vi "Send Display Settings to Analyze Actor.vi"(8 "error in (no error)":errorcluster, 11 "AF IMAQ Display in":refnum<class "HIJ Vision Display.lvclass">) -> (0 "error out":errorcluster, 3 "AF IMAQ Display out":refnum<class "HIJ Vision Display.lvclass">)   [LabVIEW 2020, in "HIJ Vision Display.lvlib" / "HIJ Vision Display.lvclass"]
uses:
  HIJ Vision Display.lvclass
  HIJ Vision Display.lvclass/HIJ Vision Display.ctl
  Analyze/Analyze Parameter/Analyze Parameter Calibration/Analyze Parameter Calibration.lvclass
  C:/POLARIS Programme/POLARIS-AS-3-Cams/Submodules/HIJ Vision/Analyze/Analyze Parameter/Analyze Parameter Base/Analyze Parameter Base.lvclass
  Analyze/Analyze Parameter/Analyze Parameter ROI/Analyze Parameter ROI.lvclass
  Analyze/Analyze Parameter/Analyze Parameter ROI/Analyze Parameter ROI.lvclass/Analyze Parameter ROI.ctl
  Analyze/Analyze Actor/Analyze Actor Messages/Set Analyze Parameter Msg/Set Analyze Parameter Msg.lvclass/Set Analyze Parameter Msg.ctl
  <vilib>/ActorFramework/Message Enqueuer/Message Enqueuer.lvclass/Message Enqueuer.ctl
  Analyze/Analyze Parameter/Analyze Parameter Calibration/Analyze Parameter Calibration.lvclass/Analyze Parameter Calibration.ctl
  Analyze/Analyze Parameter/Analyze Parameter ROI/Write ROI Descriptor.vi
  Analyze/Analyze Parameter/Analyze Parameter Calibration/Write Calibration.vi
  <vilib>/ActorFramework/Message Enqueuer/Enqueue.vi
  Analyze/Analyze Actor/Analyze Actor Messages/Set Analyze Parameter Msg/Set Analyze Parameter Msg.lvclass
  C:/Program Files (x86)/National Instruments/LabVIEW 2020/vi.lib/ActorFramework/Message/Message.lvclass
  <vilib>/ActorFramework/Message Priority Queue/Priority Enqueue.vi
  <vilib>/ActorFramework/Message Enqueuer/Message Enqueuer.lvclass
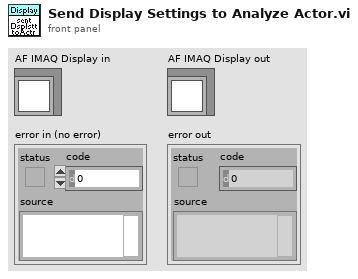
[diagram p1: front panel]
types:
  T1 = typedef "ROI Descriptor" = cluster{"Global Rectangle":i32[], "Contours":cluster{"ID":enum32{"External", "Internal"}, "Type":u32, "Coordinates":i32[]}[]}
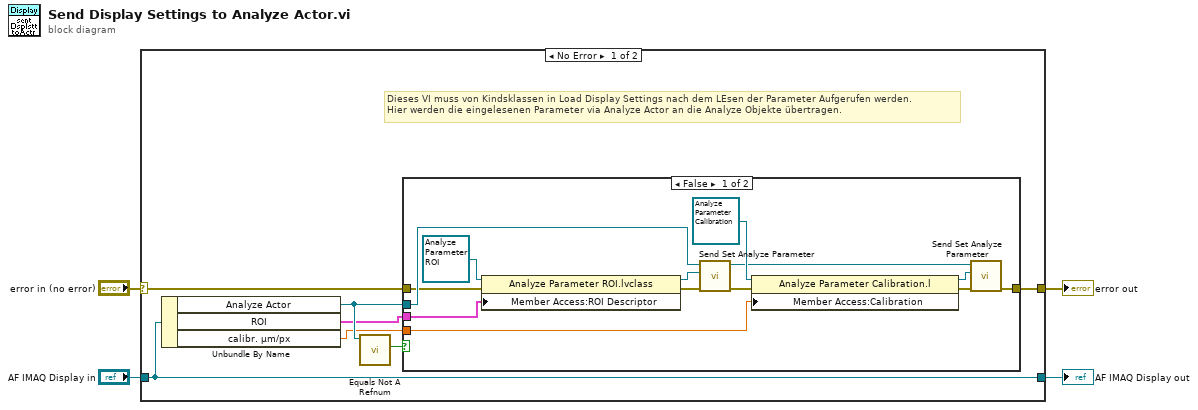
[diagram p0: block diagram]
diagram:
  n1 = case shown="No Error" "error in (no error)" {
    selector: "error in (no error)" -> [w5 w27]
    tunnel: "AF IMAQ Display in" -> [w7 w26]
    tunnel: [w7 w26] -> w3
    tunnel: [w6 w27] -> w2
    frame No Error {
      # "Dieses VI muss von Kindsklassen in Load Display Settings nach dem LEsen der Parameter Aufgerufen werden.\nHier werden die eingelesenen Parameter via Analyze Actor an die Analyze Objekte übertragen."
      n2 = Unbundle By Name(w7) -> ("Analyze Actor"=w10:refnum<class "Message Enqueuer.lvclass">, "ROI"=w8:T1, "calibr. µm/px"=w9:sgl[unit])
      n3 = call <vilib>:"Equals Not A Refnum.vi"("Message Enqueuer"=w10) -> ("Not a refnum?"=w11:bool)  [unwired: 10 in]
      n4 = case shown="False" w11 {
        tunnel: w10 -> [w24 _]
        tunnel: w9 -> [w22 _]
        tunnel: w8 -> [w18 _]
        tunnel: w5 -> [w16 w25]
        tunnel: [w12 w25] -> w6
        frame False {
          n5 = property class="Analyze Parameter ROI.lvclass"(reference=refnum<class "Analyze Parameter ROI.lvclass"> refnum ("Analyze Parameter ROI.lvclass"), error in=w16, "Member Access:ROI Descriptor"=w18) -> (reference out=w17:refnum<class "Analyze Parameter ROI.lvclass">, error out=w15:errorcluster)
          n6 = call "Send Set Analyze Parameter.vi"("error in (no error)"=w15, "Analyze Parameter"=w17, "Message Enqueuer"=w24) -> ("error out"=w14:errorcluster, "Message Enqueuer out"=w20:refnum<class "Message Enqueuer.lvclass">)  [unwired: 7 in]
          n7 = property class="Analyze Parameter Calibration.l"(reference=refnum<class "Analyze Parameter Calibration.lvclass"> refnum ("Analyze Parameter Calibration.lvclass"), error in=w14, "Member Access:Calibration"=w22) -> (reference out=w21:refnum<class "Analyze Parameter Calibration.lvclass">, error out=w13:errorcluster)
          n8 = call "Send Set Analyze Parameter.vi"("error in (no error)"=w13, "Analyze Parameter"=w21, "Message Enqueuer"=w20) -> ("error out"=w12:errorcluster)  [unwired: 7 in, 1 out]
        }
        frame True {
        }
      }
    }
    frame Error {
    }
  }
  "error out" <- w2
  "AF IMAQ Display out" <- w3
